vi "SpreadsheetRead.vi"() -> (2 "Output Cluster":cluster{"X Array":dbl[], "Y Array":dbl[]}={"X Array"=[0.0, 0.001, 0.002, 0.003, 0.004, 0.005, 0.006, 0.007, 0.008, 0.009, 0.01, 0.011, 0.012, 0.013, 0.014, 0.015, 0.016, 0.017, 0.018, 0.019, 0.02, 0.021, 0.022, 0.023, 0.024, 0.025, 0.026, 0.027, 0.028, 0.029, 0.03, 0.031, 0.032, 0.033, 0.034, 0.035, 0.036, 0.037, 0.038, 0.039, 0.04, 0.041, 0.042, 0.043, 0.044, 0.045, 0.046, 0.047, 0.048, 0.049, 0.05, 0.051, 0.052, 0.053, 0.054, 0.055, 0.056, 0.057, 0.058, 0.059, 0.06, 0.061, 0.062, 0.063, 0.064, 0.065, 0.066, 0.067, 0.068, 0.069, 0.07, 0.071, 0.072, 0.073, 0.074, 0.075, 0.076, 0.077, 0.078, 0.079, 0.08, 0.081, 0.082, 0.083, 0.084, 0.085, 0.086, 0.087, 0.088, 0.089, 0.09, 0.091, 0.092, 0.093, 0.094, 0.095, 0.096, 0.097, 0.098, 0.099], "Y Array"=[0.0, 1.545, 2.939, 4.045, 4.755, 5.0, 4.755, 4.045, 2.939, 1.545, 0.0, -1.545, -2.939, -4.045, -4.755, -5.0, -4.755, -4.045, -2.939, -1.545, -0.0, 1.545, 2.939, 4.045, 4.755, 5.0, 4.755, 4.045, 2.939, 1.545, 0.0, -1.545, -2.939, -4.045, -4.755, -5.0, -4.755, -4.045, -2.939, -1.545, -0.0, 1.545, 2.939, 4.045, 4.755, 5.0, 4.755, 4.045, 2.939, 1.545, -0.0, -1.545, -2.939, -4.045, -4.755, -5.0, -4.755, -4.045, -2.939, -1.545, -0.0, 1.545, 2.939, 4.045, 4.755, 5.0, 4.755, 4.045, 2.939, 1.545, -0.0, -1.545, -2.939, -4.045, -4.755, -5.0, -4.755, -4.045, -2.939, -1.545, -0.0, 1.545, 2.939, 4.045, 4.755, 5.0, 4.755, 4.045, 2.939, 1.545, 0.0, -1.545, -2.939, -4.045, -4.755, -5.0, -4.755, -4.045, -2.939, -1.545]} {"Y Array" format="%#_13g"; "X Array" format="%#_13g"})   [LabVIEW 2015]
uses:
  <vilib>/Utility/file.llb/Read Delimited Spreadsheet (DBL).vi
panel:
  out "Spreadsheet Waveform":cluster{"all rows":dbl[], "all rows":dbl[]}(graph)={"all rows"=[0.0, 0.001, 0.002, 0.003, 0.004, 0.005, 0.006, 0.007, 0.008, 0.009, 0.01, 0.011, 0.012, 0.013, 0.014, 0.015, 0.016, 0.017, 0.018, 0.019, 0.02, 0.021, 0.022, 0.023, 0.024, 0.025, 0.026, 0.027, 0.028, 0.029, 0.03, 0.031, 0.032, 0.033, 0.034, 0.035, 0.036, 0.037, 0.038, 0.039, 0.04, 0.041, 0.042, 0.043, 0.044, 0.045, 0.046, 0.047, 0.048, 0.049, 0.05, 0.051, 0.052, 0.053, 0.054, 0.055, 0.056, 0.057, 0.058, 0.059, 0.06, 0.061, 0.062, 0.063, 0.064, 0.065, 0.066, 0.067, 0.068, 0.069, 0.07, 0.071, 0.072, 0.073, 0.074, 0.075, 0.076, 0.077, 0.078, 0.079, 0.08, 0.081, 0.082, 0.083, 0.084, 0.085, 0.086, 0.087, 0.088, 0.089, 0.09, 0.091, 0.092, 0.093, 0.094, 0.095, 0.096, 0.097, 0.098, 0.099], "all rows"=[0.0, 1.545, 2.939, 4.045, 4.755, 5.0, 4.755, 4.045, 2.939, 1.545, 0.0, -1.545, -2.939, -4.045, -4.755, -5.0, -4.755, -4.045, -2.939, -1.545, -0.0, 1.545, 2.939, 4.045, 4.755, 5.0, 4.755, 4.045, 2.939, 1.545, 0.0, -1.545, -2.939, -4.045, -4.755, -5.0, -4.755, -4.045, -2.939, -1.545, -0.0, 1.545, 2.939, 4.045, 4.755, 5.0, 4.755, 4.045, 2.939, 1.545, -0.0, -1.545, -2.939, -4.045, -4.755, -5.0, -4.755, -4.045, -2.939, -1.545, -0.0, 1.545, 2.939, 4.045, 4.755, 5.0, 4.755, 4.045, 2.939, 1.545, -0.0, -1.545, -2.939, -4.045, -4.755, -5.0, -4.755, -4.045, -2.939, -1.545, -0.0, 1.545, 2.939, 4.045, 4.755, 5.0, 4.755, 4.045, 2.939, 1.545, 0.0, -1.545, -2.939, -4.045, -4.755, -5.0, -4.755, -4.045, -2.939, -1.545]}
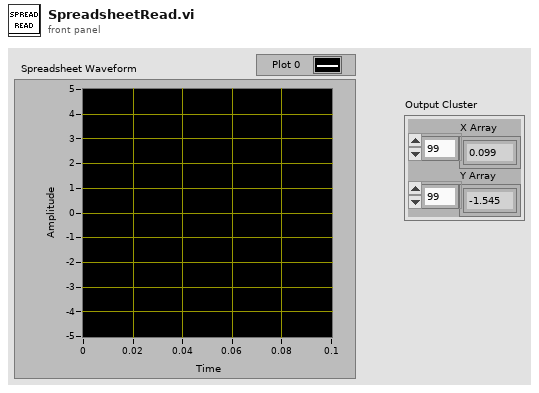
[diagram p1: front panel]
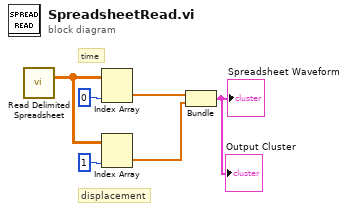
[diagram p0: block diagram]
diagram:
  # "displacement"
  # "time"
  n1 = call-poly <vilib>:"Read Delimited Spreadsheet.vi"() -> ("all rows"=w6:dbl[][])  [unwired: 10 in, 5 out]
  n2 = Index Array(array=w6, index (col)=0) -> (element=w3:dbl[])  [unwired: 1 in]
  n3 = Index Array(array=w6, index (col)=1) -> (element=w2:dbl[])  [unwired: 1 in]
  n4 = Bundle("all rows"=w3, "all rows"=w2) -> (→"Spreadsheet Waveform" →"Output Cluster":cluster{"all rows":dbl[], "all rows":dbl[]})  [unwired: 1 in]
